vi "Shutdown PS2.vi"(6 "Current Limit (0)":dbl min=0.0 max=6.0 format="%#.2g", 8 "error in (no error)":errorcluster, 9 "Output Voltage (0)":dbl min=0.0 max=18.0 format="%#.2f", 10 "Maximum Output Voltage (0)":dbl min=0.0 max=72.0 format="%#.2f", 11 "PS 2":refnum<visa-resource-name>) -> (0 "error out":errorcluster)   [LabVIEW 2015]
uses:
  <instrlib>/BK Precision 178XB Series/BK Precision 178XB Series.lvlib
panel:
  # "Initialize \"Battery\" PS"
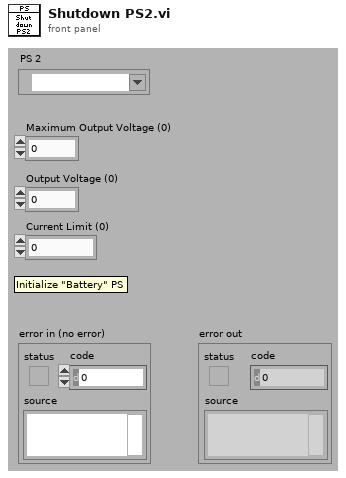
[diagram p1: front panel]
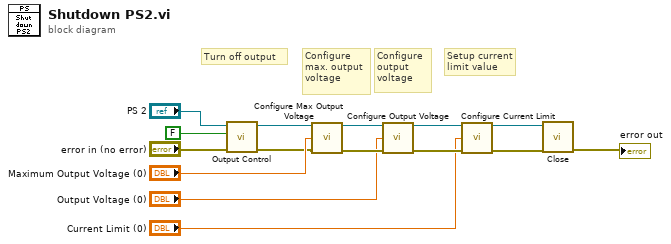
[diagram p0: block diagram]
diagram:
  # "Setup current\nlimit value"
  # "Configure output\nvoltage"
  # "Configure\nmax. output\nvoltage"
  # "Turn off output"
  n1 = call <instrlib>:"Output Control.vi"("error in (no error)"="error in (no error)", "Enable Output Terminals (F: Off)"=FALSE, "VISA resource name"="PS 2") -> ("error out"=w6:errorcluster, "VISA resource name out"=w7:refnum<visa-resource-name>)  [unwired: 7 in]
  n2 = call <instrlib>:"Configure Max Output Voltage.vi"("VISA resource name"=w7, "Maximum Output Voltage (18)"="Maximum Output Voltage (0)", "error in (no error)"=w6) -> ("VISA resource name out"=w14:refnum<visa-resource-name>, "error out"=w11:errorcluster)  [unwired: 11 in]
  n3 = call <instrlib>:"Configure Output Voltage.vi"("VISA resource name"=w14, "Output Voltage (0)"="Output Voltage (0)", "error in (no error)"=w11) -> ("VISA resource name out"=w13:refnum<visa-resource-name>, "error out"=w12:errorcluster)  [unwired: 11 in]
  n4 = call <instrlib>:"Configure Current Limit.vi"("VISA resource name"=w13, "Current Limit (0)"="Current Limit (0)", "error in (no error)"=w12) -> ("VISA resource name out"=w2:refnum<visa-resource-name>, "error out"=w4:errorcluster)  [unwired: 11 in]
  n5 = call <instrlib>:"Close.vi"("error in (no error)"=w4, "VISA resource name"=w2) -> ("error out"=→"error out":errorcluster)  [unwired: 9 in]
